vi "ReadDataFromLabVIEWINI.vi"(8 "error in (no error)":errorcluster, 11 "DNL_Font":refnum<vi>) -> (0 "error out":errorcluster={"status"=TRUE, "code"=1055, "source"="Property Node in Windows.vi->Populate Font ComboBox.vi->Populate Font Control.vi->ReadDataFromLabVIEWINI.vi"}, 3 "INI Data":T1={"Show Layer Tab?"=FALSE, "Show Terminals?"=FALSE, "Text"={"Font"="Small Fonts", "Alignment"=0, "Size"=9}, "3rd party Templates"={"Store 3rd party Templates?"=TRUE, "Folder Name"="3rd party"}, "Merge user layers on commit"=TRUE, "Body Text"={"Line 1 text"="", "Line 2 text"="", "Line 3 text"="", "Line 4 text"="", "Line 1 color"=0, "Line 2 color"=0, "Line 3 color"=0, "Line 4 color"=0, "Body Text Spec"={"Font"="", "Alignment"=0, "Size"=3}, "Center text vertically"=FALSE, "Capitalize Text"=FALSE}, "Fill Color"=16711680, "Edge Color"=0, "Tab"=0, "Tool"=enum."Ellipse", "Disable Layers?"=FALSE} {"Body Text"."Body Text Spec"."Alignment" items=["left", "center", "right"]; "Text"."Alignment" items=["left", "center", "right"]})   [LabVIEW 2012]
uses:
  <resource>/plugins/NIIconEditor/Controls/INI.ctl
  <vilib>/LabVIEW Icon API/lv_icon/Controls/Font.ctl
  <vilib>/LabVIEW Icon API/lv_icon/Controls/Alignment.ctl
  <resource>/plugins/NIIconEditor/Controls/Font Size.ctl
  <vilib>/LabVIEW Icon API/lv_icon/Controls/BodyText.ctl
  <vilib>/LabVIEW Icon API/lv_icon/Controls/IEColor.ctl
  <resource>/plugins/NIIconEditor/Controls/Tools.ctl
  <resource>/plugins/NIIconEditor/Controls/Pen.ctl
  <resource>/plugins/NIIconEditor/Controls/Line.ctl
  <resource>/plugins/NIIconEditor/Controls/Dropper.ctl
  <resource>/plugins/NIIconEditor/Controls/Fill.ctl
  <resource>/plugins/NIIconEditor/Controls/IERect.ctl
  <resource>/plugins/NIIconEditor/Controls/FRect.ctl
  <resource>/plugins/NIIconEditor/Controls/Circle.ctl
  <resource>/plugins/NIIconEditor/Controls/FCircle.ctl
  <resource>/plugins/NIIconEditor/Controls/Rubber.ctl
  <resource>/plugins/NIIconEditor/Controls/Text.ctl
  <resource>/plugins/NIIconEditor/Controls/Selection.ctl
  <resource>/plugins/NIIconEditor/Controls/Move.ctl
  <resource>/dialog/lvconfig.llb/LV Config Read String.vi
  <resource>/dialog/lvconfig.llb/LV Config Read Color.vi
  <resource>/dialog/lvconfig.llb/LV Config Read Boolean.vi
panel:
  in  "INI Data":T1={"Show Layer Tab?"=TRUE, "Show Terminals?"=FALSE, "Text"={"Font"="Small Fonts", "Alignment"=1, "Size"=9}, "3rd party Templates"={"Store 3rd party Templates?"=TRUE, "Folder Name"="3rd party"}, "Merge user layers on commit"=FALSE, "Body Text"={"Line 1 text"="", "Line 2 text"="", "Line 3 text"="", "Line 4 text"="", "Line 1 color"=0, "Line 2 color"=0, "Line 3 color"=0, "Line 4 color"=0, "Body Text Spec"={"Font"="Small Fonts", "Alignment"=1, "Size"=9}, "Center text vertically"=TRUE, "Capitalize Text"=TRUE}, "Fill Color"=16711680, "Edge Color"=0, "Tab"=0, "Tool"=enum."Pencil", "Disable Layers?"=FALSE} {"Body Text"."Body Text Spec"."Alignment" items=["left", "center", "right"]; "Text"."Alignment" items=["left", "center", "right"]}
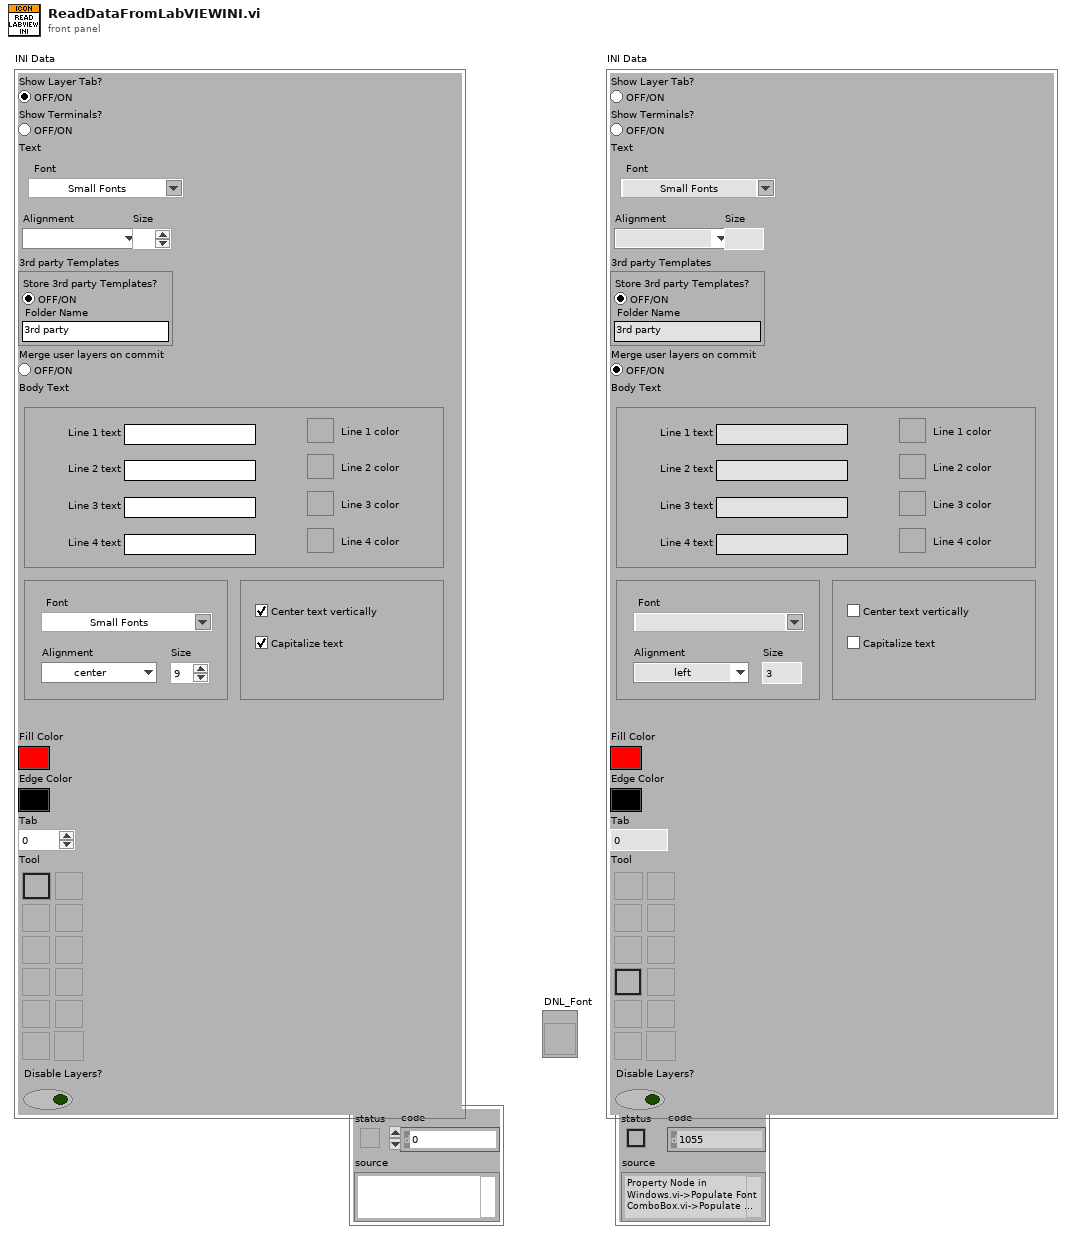
[diagram p1: front panel]
types:
  T1 = typedef "INI.ctl" = cluster{"Show Layer Tab?":bool, "Show Terminals?":bool, "Text":cluster{"Font":T2, "Alignment":T3, "Size":T4}, "3rd party Templates":cluster{"Store 3rd party Templates?":bool, "Folder Name":string}, "Merge user layers on commit":bool, "Body Text":T5, "Fill Color":T6, "Edge Color":T6, "Tab":u16, "Tool":T7, "Disable Layers?":bool}
  T2 = typedef "Font.ctl" = string
  T3 = typedef "Alignment.ctl" = u16
  T4 = typedef "Font Size.ctl" = u8
  T5 = typedef "BodyText.ctl" = cluster{"Line 1 text":string, "Line 2 text":string, "Line 3 text":string, "Line 4 text":string, "Line 1 color":u32, "Line 2 color":u32, "Line 3 color":u32, "Line 4 color":u32, "Body Text Spec":cluster{"Font":T2, "Alignment":T3, "Size":u8}, "Center text vertically":bool, "Capitalize Text":bool}
  T6 = typedef "IEColor.ctl" = u32
  T7 = typedef "Tools.ctl" = enum32{"Pencil", "Line", "Dropper", "Fill", "Rectangle", "Filled Rectangle", "Ellipse", "Filled Ellipse", "Eraser", "Text", "Select", "Move"}
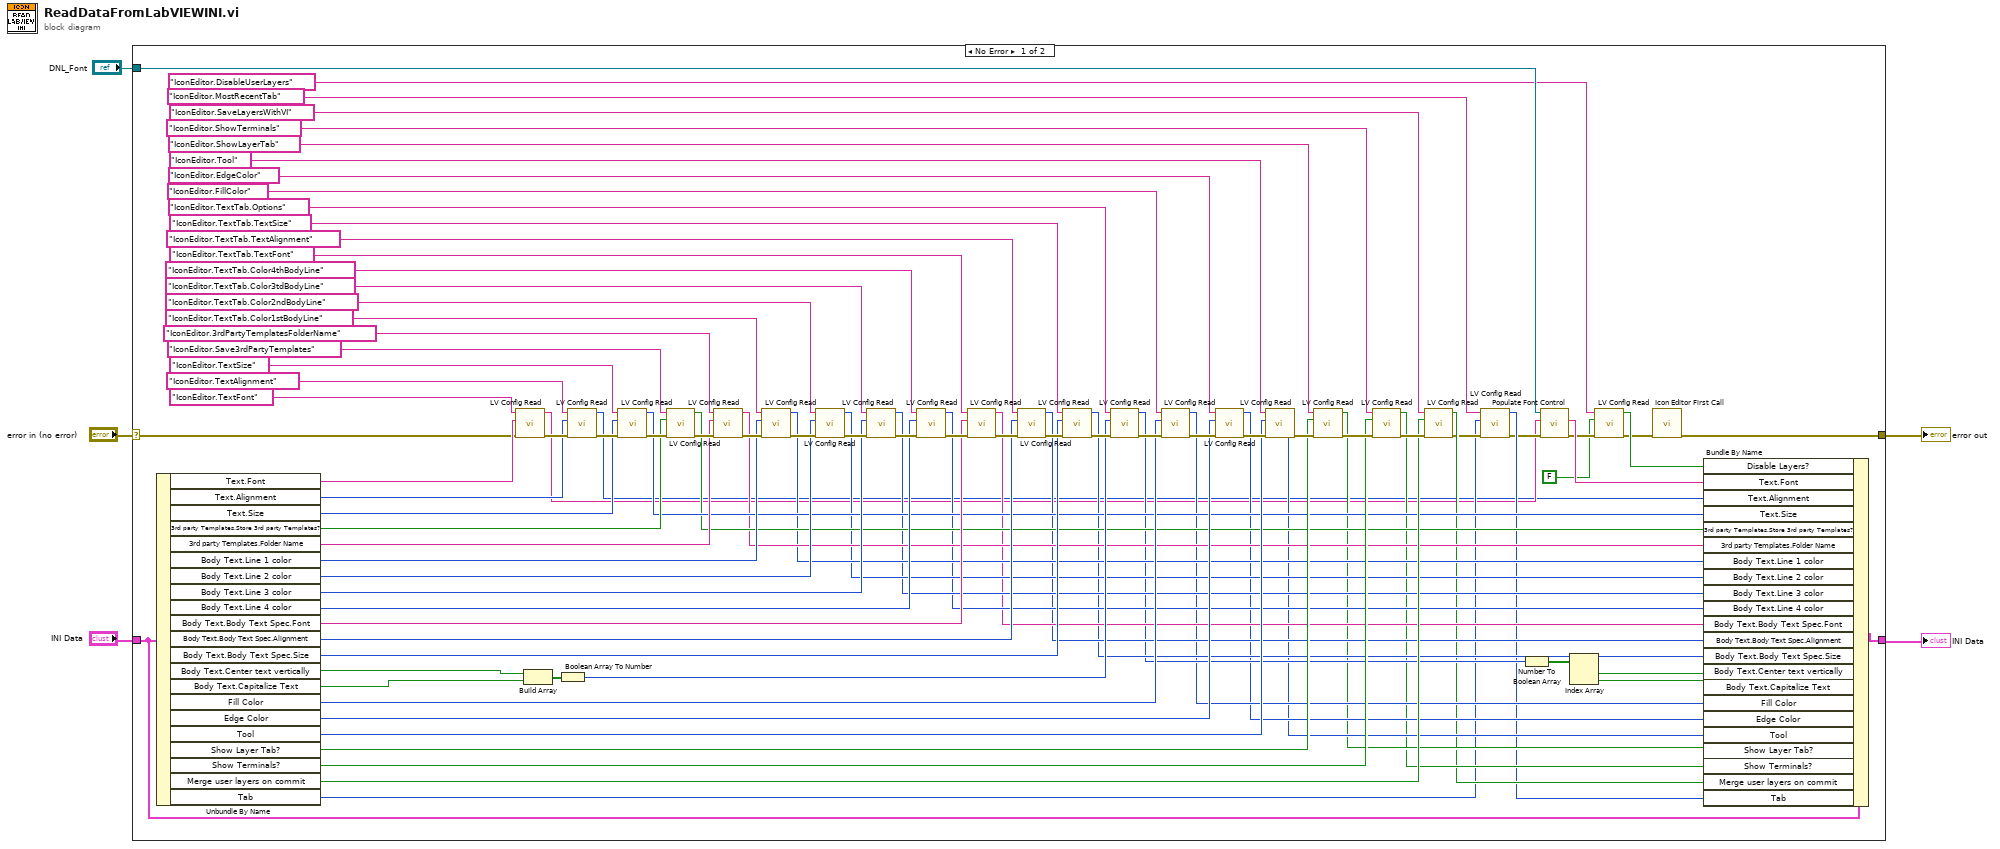
[diagram p0: block diagram]
diagram:
  n1 = case shown="No Error" "error in (no error)" {
    selector: "error in (no error)" -> [w17 w103]
    tunnel: [w11 w103] -> w4
    tunnel: "INI Data" -> [w24 _]
    tunnel: [w25 _] -> w3
    tunnel: "DNL_Font" -> [w12 _]
    frame No Error {
      n2 = Unbundle By Name(w24) -> ("Text.Font"=w65:T2, "Text.Alignment"=w64:T3, "Text.Size"=w63:T4, "3rd party Templates.Store 3rd party Templates?"=w62:bool, "3rd party Templates.Folder Name"=w58:string, "Body Text.Line 1 color"=w57:u32, "Body Text.Line 2 color"=w56:u32, "Body Text.Line 3 color"=w55:u32, "Body Text.Line 4 color"=w54:u32, "Body Text.Body Text Spec.Font"=w53:T2, "Body Text.Body Text Spec.Alignment"=w52:T3, "Body Text.Body Text Spec.Size"=w51:u8, "Body Text.Center text vertically"=w59:bool, "Body Text.Capitalize Text"=w60:bool, "Fill Color"=w49:T6, "Edge Color"=w48:T6, "Tool"=w47:T7, "Show Layer Tab?"=w46:bool, "Show Terminals?"=w45:bool, "Merge user layers on commit"=w44:bool, "Tab"=w21:u16)
      n3 = call-poly <resource>:"LV Config Read.vi"("error in"=w17, "default value"=w65, "key"="IconEditor.TextFont") -> ("error out"=w102:errorcluster, "value"=w18:string)  [unwired: 3 out]
      n4 = Build Array(w59, w60) -> (w61:bool[])
      n5 = Boolean Array To Number(Boolean array=w61) -> (number=w50:u32)
      n6 = call-poly <resource>:"LV Config Read.vi"("error in"=w102, "default value"=w64, "key"="IconEditor.TextAlignment") -> ("error out"=w101:errorcluster, "value"=w14:u32)  [unwired: 3 out]
      n7 = call-poly <resource>:"LV Config Read.vi"("error in"=w101, "default value"=w63, "key"="IconEditor.TextSize") -> ("error out"=w100:errorcluster, "value"=w43:u32)  [unwired: 3 out]
      n8 = call-poly <resource>:"LV Config Read.vi"("error in"=w100, "default value"=w62, "key"="IconEditor.Save3rdPartyTemplates") -> ("error out"=w99:errorcluster, "value"=w42:bool)  [unwired: 3 out]
      n9 = call-poly <resource>:"LV Config Read.vi"("error in"=w99, "default value"=w58, "key"="IconEditor.3rdPartyTemplatesFolderName") -> ("error out"=w98:errorcluster, "value"=w41:string)  [unwired: 3 out]
      n10 = call-poly <resource>:"LV Config Read.vi"("error in"=w98, "default value"=w57, "key"="IconEditor.TextTab.Color1stBodyLine") -> ("error out"=w97:errorcluster, "value"=w40:u32)  [unwired: 3 out]
      n11 = call-poly <resource>:"LV Config Read.vi"("error in"=w97, "default value"=w56, "key"="IconEditor.TextTab.Color2ndBodyLine") -> ("error out"=w96:errorcluster, "value"=w39:u32)  [unwired: 3 out]
      n12 = call-poly <resource>:"LV Config Read.vi"("error in"=w96, "default value"=w55, "key"="IconEditor.TextTab.Color3tdBodyLine") -> ("error out"=w95:errorcluster, "value"=w38:u32)  [unwired: 3 out]
      n13 = call-poly <resource>:"LV Config Read.vi"("error in"=w95, "default value"=w54, "key"="IconEditor.TextTab.Color4thBodyLine") -> ("error out"=w94:errorcluster, "value"=w37:u32)  [unwired: 3 out]
      n14 = call-poly <resource>:"LV Config Read.vi"("error in"=w94, "default value"=w53, "key"="IconEditor.TextTab.TextFont") -> ("error out"=w93:errorcluster, "value"=w36:string)  [unwired: 3 out]
      n15 = call-poly <resource>:"LV Config Read.vi"("error in"=w93, "default value"=w52, "key"="IconEditor.TextTab.TextAlignment") -> ("error out"=w92:errorcluster, "value"=w35:u32)  [unwired: 3 out]
      n16 = call-poly <resource>:"LV Config Read.vi"("error in"=w92, "default value"=w51, "key"="IconEditor.TextTab.TextSize") -> ("error out"=w91:errorcluster, "value"=w34:u32)  [unwired: 3 out]
      n17 = call-poly <resource>:"LV Config Read.vi"("error in"=w91, "default value"=w50, "key"="IconEditor.TextTab.Options") -> ("error out"=w90:errorcluster, "value"=w33:u32)  [unwired: 3 out]
      n18 = call-poly <resource>:"LV Config Read.vi"("error in"=w90, "default value"=w49, "key"="IconEditor.FillColor") -> ("error out"=w89:errorcluster, "value"=w31:u32)  [unwired: 3 out]
      n19 = call-poly <resource>:"LV Config Read.vi"("error in"=w89, "default value"=w48, "key"="IconEditor.EdgeColor") -> ("error out"=w88:errorcluster, "value"=w30:u32)  [unwired: 3 out]
      n20 = call-poly <resource>:"LV Config Read.vi"("error in"=w88, "default value"=w47, "key"="IconEditor.Tool") -> ("error out"=w87:errorcluster, "value"=w29:u32)  [unwired: 3 out]
      n21 = call-poly <resource>:"LV Config Read.vi"("error in"=w87, "default value"=w46, "key"="IconEditor.ShowLayerTab") -> ("error out"=w86:errorcluster, "value"=w28:bool)  [unwired: 3 out]
      n22 = call-poly <resource>:"LV Config Read.vi"("error in"=w86, "default value"=w45, "key"="IconEditor.ShowTerminals") -> ("error out"=w67:errorcluster, "value"=w27:bool)  [unwired: 3 out]
      n23 = call-poly <resource>:"LV Config Read.vi"("error in"=w67, "default value"=w44, "key"="IconEditor.SaveLayersWithVI") -> ("error out"=w23:errorcluster, "value"=w26:bool)  [unwired: 3 out]
      n24 = call-poly <resource>:"LV Config Read.vi"("error in"=w23, "default value"=w21, "key"="IconEditor.MostRecentTab") -> ("error out"=w19:errorcluster, "value"=w20:u32)  [unwired: 3 out]
      n25 = Number To Boolean Array(number=w33) -> (Boolean array=w32:bool[])
      n26 = call <resource>:"Populate Font Control.vi"("error in (no error)"=w19, "Font in"=w18, "DNL_Font"=w12) -> ("error out"=w10:errorcluster, "Font out"=w13:string)  [unwired: 7 out]
      n27 = Index Array(array=w32) -> (element #1=w16:bool, element #2=w15:bool)  [unwired: 2 in]
      n28 = call-poly <resource>:"LV Config Read.vi"("error in"=w10, "default value"=FALSE ("value"), "key"="IconEditor.DisableUserLayers") -> ("error out"=w6:errorcluster, "value"=w8:bool)  [unwired: 1 in, 2 out]
      n29 = call <resource>:"Icon Editor First Call.vi"("error in (no error)"=w6) -> ("error out"=w11:errorcluster)  [unwired: 10 out]
      n30 = Bundle By Name(cluster=w24, "Disable Layers?"=w8, "Text.Font"=w13, "Text.Alignment"=w14, "Text.Size"=w43, "3rd party Templates.Store 3rd party Templates?"=w42, "3rd party Templates.Folder Name"=w41, "Body Text.Line 1 color"=w40, "Body Text.Line 2 color"=w39, "Body Text.Line 3 color"=w38, "Body Text.Line 4 color"=w37, "Body Text.Body Text Spec.Font"=w36, "Body Text.Body Text Spec.Alignment"=w35, "Body Text.Body Text Spec.Size"=w34, "Body Text.Center text vertically"=w16, "Body Text.Capitalize Text"=w15, "Fill Color"=w31, "Edge Color"=w30, "Tool"=w29, "Show Layer Tab?"=w28, "Show Terminals?"=w27, "Merge user layers on commit"=w26, "Tab"=w20) -> (w25:T1)
    }
    frame Error {
    }
  }
  "error out" <- w4
  "INI Data" <- w3
